vi "GenericDriveIO.vi"(0 "GenericDriveCommand":T2="DePowerMotor", 2 "Channel Name":string, 4 "String Value":string, 6 "Numeric Value":dbl format="%.2f", 8 "Address":u8, 9 "Type":T1, 10 "Port Name":string) -> (3 "Error Description":string, 5 "String Reply":string, 7 "Numeric Reply":sgl format="%.2f")   [LabVIEW 2022 SP3]
uses:
  GenericDriveCommand.ctl
  Traverse Type.ctl
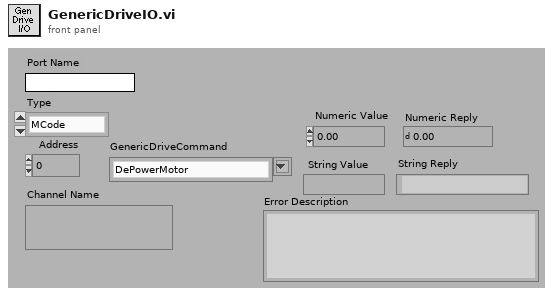
[diagram p1: front panel]
types:
  T1 = typedef "Traverse Type.ctl" = enum16{"MCode", "Dynamixel"}
  T2 = typedef "GenericDriveCommand.ctl" = string
  T3 = typedef "Dynamixel Commands.ctl" = enum16{"Torque Enable", "Present Position", "Threshold", "Max Position Limit", "Acceleration Profile", "Velocity Profile", "Goal Position", "Position Proportional Gain", "Position Integral Gain", "Position Differential Gain ", "Shutdown", "Write Operating Mode", "Read Operating Mode"}
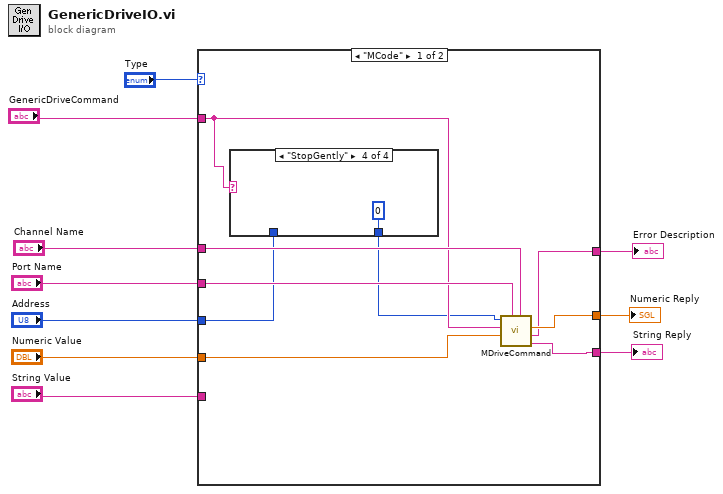
[diagram p0: block diagram]
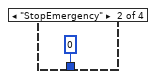
[diagram p3: hidden frame]
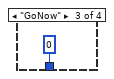
[diagram p4: hidden frame]
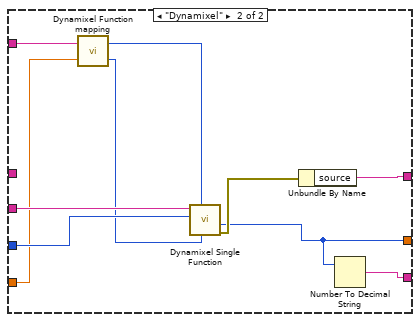
[diagram p5: hidden frame]
diagram:
  n1 = case shown="\"MCode\"" "Type" {
    tunnel: "Port Name" -> [w18 w33]
    tunnel: "Address" -> [w12 w32]
    tunnel: "Numeric Value" -> [w17 w25]
    tunnel: "String Value" -> [_ _]
    tunnel: "Channel Name" -> [w19 _]
    tunnel: [w16 w29] -> w5
    tunnel: [w15 w28] -> w4
    tunnel: "GenericDriveCommand" -> [w13 w27]
    tunnel: [w14 w30] -> w1
    frame "MCode" {
      n2 = case shown="\"StopGently\"" w13 {
        tunnel: w12 -> [w20 _ _ _]
        tunnel: [w20 u8 0 ("Address") u8 0 ("Address") u8 0 ("Address")] -> w11
        frame Default {
        }
        frame "StopEmergency" {
        }
        frame "GoNow" {
        }
        frame "StopGently" {
        }
      }
      n3 = call "MDriveCommand.vi"("Channel Name"=w19, "Port Name"=w18, "Numeric Value"=w17, "MDriveCommand"=w13, "Address"=w11) -> ("String Reply"=w15:string, "Error Description"=w14:string, "Numeric Reply"=w16:dbl)  [unwired: 2 in, 1 out]
    }
    frame "Dynamixel" {
      n4 = call "Dynamixel Function mapping.vi"("data In"=w25, "GenericDriveCommand"=w27) -> ("data Out"=w24:u32, "Function"=w26:T3)
      n5 = call "Dynamixel Single Function.vi"("data"=w24, "Function"=w26, "dynamixel_id"=w32, "Com port"=w33) -> ("error out"=w31:errorcluster, "function return"=w29:i32)  [unwired: 6 in]
      n6 = Unbundle By Name(w31) -> ("source"=w30:string)
      n7 = Number To Decimal String(number=w29) -> (decimal integer string=w28:string)  [unwired: 1 in]
    }
  }
  "String Reply" <- w4
  "Numeric Reply" <- w5
  "Error Description" <- w1
